vi "Project.vi"() -> ()   [LabVIEW 2023]
uses:
  <vilib>/DAQmx/read.llb/DAQmx Read (Digital Bool 1Line 1Point).vi
  <vilib>/DAQmx/write.llb/DAQmx Write (Digital Bool 1Line 1Point).vi
  <vilib>/DAQmx/read.llb/DAQmx Read (Digital 1D Bool NChan 1Samp 1Line).vi
  <vilib>/DAQmx/create/channels.llb/DAQmx Create Channel (DO-Digital Output).vi
  <vilib>/DAQmx/create/channels.llb/DAQmx Create Channel (DI-Digital Input).vi
  <vilib>/DAQmx/miscellaneous.llb/DAQmx Fill In Error Info.vi
panel:
  in  "Cry":tag
  in  "Motor":tag
  in  "Available":tag
  in  "Fan":tag
  in  "Wet":tag
  in  "Buzzer":tag
  in  "stop":bool
  out "Cry":bool
  out "Available":bool
  out "Wet":bool
  # "Indication Panel"
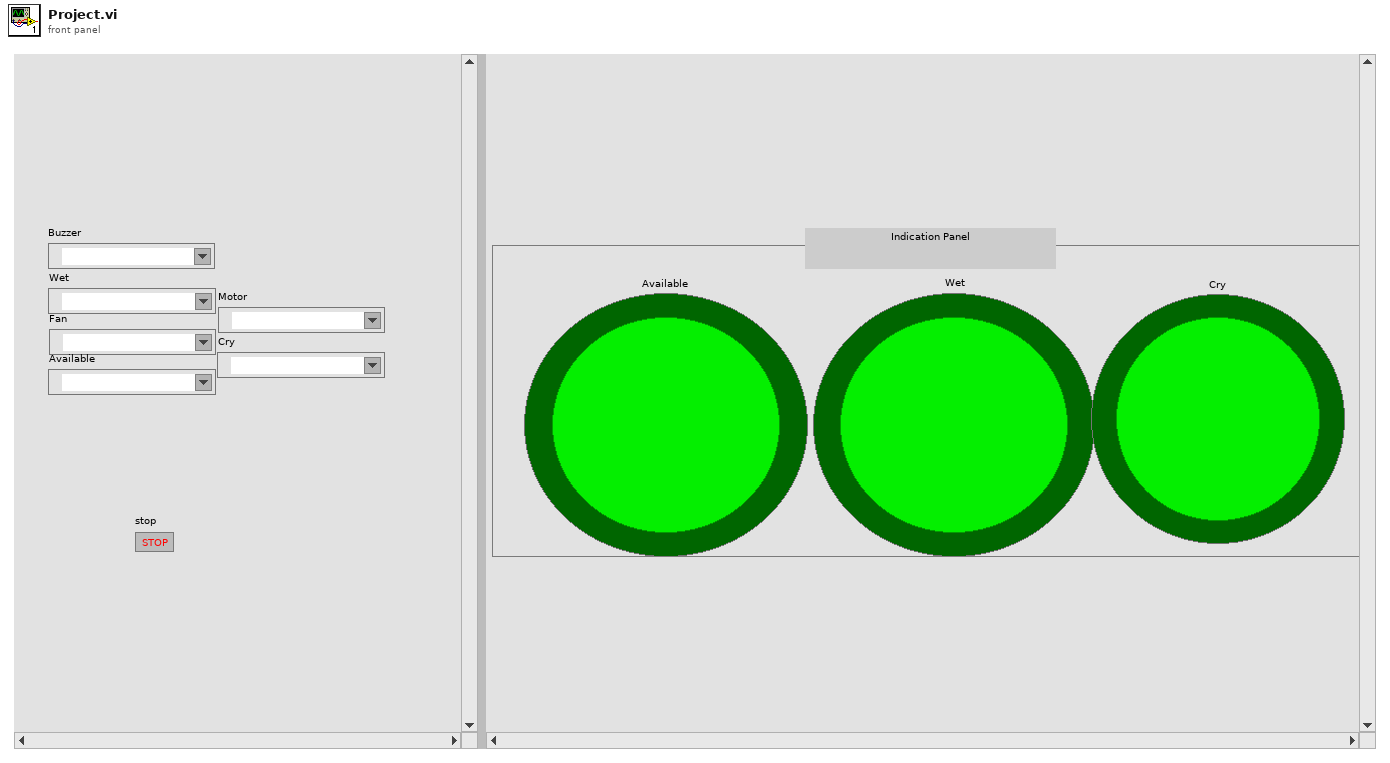
[diagram p1: front panel]
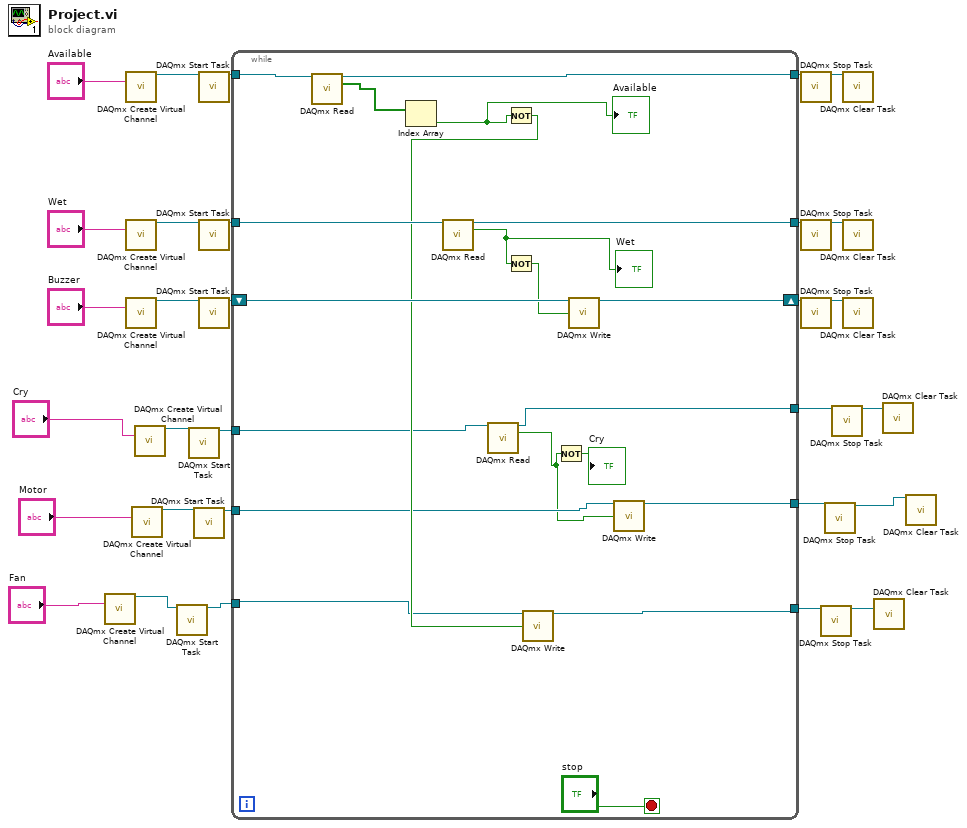
[diagram p0: block diagram]
diagram:
  n1 = call-poly <vilib>:"DAQmx Create Virtual Channel.vi"("lines"="Fan") -> ("task out"=w15:refnum<k21>)  [unwired: 13 in, 1 out]
  n2 = call-poly <vilib>:"DAQmx Create Virtual Channel.vi"("lines"="Available") -> ("task out"=w12:refnum<k21>)  [unwired: 13 in, 1 out]
  n3 = call-poly <vilib>:"DAQmx Create Virtual Channel.vi"("lines"="Wet") -> ("task out"=w24:refnum<k21>)  [unwired: 13 in, 1 out]
  n4 = call-poly <vilib>:"DAQmx Create Virtual Channel.vi"("lines"="Buzzer") -> ("task out"=w30:refnum<k21>)  [unwired: 13 in, 1 out]
  n5 = call-poly <vilib>:"DAQmx Create Virtual Channel.vi"("lines"="Motor") -> ("task out"=w6:refnum<k21>)  [unwired: 13 in, 1 out]
  n6 = call-poly <vilib>:"DAQmx Create Virtual Channel.vi"("lines"="Cry") -> ("task out"=w9:refnum<k21>)  [unwired: 13 in, 1 out]
  n7 = call <vilib>:"DAQmx Start Task.vi"("task/channels in"=w15) -> ("task out"=w14:refnum<k21>)  [unwired: 13 in, 1 out]
  n8 = call <vilib>:"DAQmx Start Task.vi"("task/channels in"=w9) -> ("task out"=w8:refnum<k21>)  [unwired: 13 in, 1 out]
  n9 = call <vilib>:"DAQmx Start Task.vi"("task/channels in"=w6) -> ("task out"=w5:refnum<k21>)  [unwired: 13 in, 1 out]
  n10 = call <vilib>:"DAQmx Start Task.vi"("task/channels in"=w12) -> ("task out"=w11:refnum<k21>)  [unwired: 13 in, 1 out]
  n11 = call <vilib>:"DAQmx Start Task.vi"("task/channels in"=w24) -> ("task out"=w23:refnum<k21>)  [unwired: 13 in, 1 out]
  n12 = call <vilib>:"DAQmx Start Task.vi"("task/channels in"=w30) -> ("task out"=w27:refnum<k21>)  [unwired: 13 in, 1 out]
  n13 = while {
    shift-right: [w50] -> w28
    shift-left: w27 -> [w49]
    tunnel: w23 -> [w47]
    tunnel: [w46] -> w22
    tunnel: [w43] -> w18
    tunnel: [w42] -> w17
    tunnel: w14 -> [w41]
    tunnel: w11 -> [w40]
    tunnel: w8 -> [w39]
    tunnel: w5 -> [w38]
    tunnel: [w37] -> w3
    tunnel: [w36] -> w1
    stop <- "stop" stop-if-true
    n14 = call-poly <vilib>:"DAQmx Read.vi"("task/channels in"=w40) -> ("task out"=w42:refnum<k21>, "data"=w35:bool[])  [unwired: 12 in, 1 out]
    n15 = Index Array(array=w35) -> (element=w34:bool)  [unwired: 1 in]
    "Available" <- w34
    n16 = call-poly <vilib>:"DAQmx Read.vi"("task/channels in"=w47) -> ("task out"=w46:refnum<k21>, "data"=w33:bool)  [unwired: 12 in, 1 out]
    "Wet" <- w33
    n17 = call-poly <vilib>:"DAQmx Read.vi"("task/channels in"=w39) -> ("task out"=w37:refnum<k21>, "data"=w31:bool)  [unwired: 12 in, 1 out]
    n18 = Not(x=w34) -> (.not. x?=w44:bool)
    n19 = Not(x=w33) -> (.not. x?=w45:bool)
    n20 = call-poly <vilib>:"DAQmx Write.vi"("task/channels in"=w41, "data"=w44) -> ("task out"=w43:refnum<k21>)  [unwired: 11 in, 2 out]
    n21 = Not(x=w31) -> (.not. x?=→"Cry":bool)
    n22 = call-poly <vilib>:"DAQmx Write.vi"("task/channels in"=w49, "data"=w45) -> ("task out"=w50:refnum<k21>)  [unwired: 11 in, 2 out]
    n23 = call-poly <vilib>:"DAQmx Write.vi"("task/channels in"=w38, "data"=w31) -> ("task out"=w36:refnum<k21>)  [unwired: 11 in, 2 out]
  }
  n24 = call <vilib>:"DAQmx Stop Task.vi"("task/channels in"=w17) -> ("task out"=w20:refnum<k21>)  [unwired: 13 in, 1 out]
  n25 = call <vilib>:"DAQmx Stop Task.vi"("task/channels in"=w22) -> ("task out"=w21:refnum<k21>)  [unwired: 13 in, 1 out]
  n26 = call <vilib>:"DAQmx Stop Task.vi"("task/channels in"=w28) -> ("task out"=w29:refnum<k21>)  [unwired: 13 in, 1 out]
  n27 = call <vilib>:"DAQmx Stop Task.vi"("task/channels in"=w18) -> ("task out"=w19:refnum<k21>)  [unwired: 13 in, 1 out]
  n28 = call <vilib>:"DAQmx Stop Task.vi"("task/channels in"=w1) -> ("task out"=w4:refnum<k21>)  [unwired: 13 in, 1 out]
  n29 = call <vilib>:"DAQmx Stop Task.vi"("task/channels in"=w3) -> ("task out"=w2:refnum<k21>)  [unwired: 13 in, 1 out]
  n30 = call <vilib>:"DAQmx Clear Task.vi"("task in"=w20) -> ()  [unwired: 14 in, 1 out]
  n31 = call <vilib>:"DAQmx Clear Task.vi"("task in"=w21) -> ()  [unwired: 14 in, 1 out]
  n32 = call <vilib>:"DAQmx Clear Task.vi"("task in"=w29) -> ()  [unwired: 14 in, 1 out]
  n33 = call <vilib>:"DAQmx Clear Task.vi"("task in"=w19) -> ()  [unwired: 14 in, 1 out]
  n34 = call <vilib>:"DAQmx Clear Task.vi"("task in"=w2) -> ()  [unwired: 14 in, 1 out]
  n35 = call <vilib>:"DAQmx Clear Task.vi"("task in"=w4) -> ()  [unwired: 14 in, 1 out]
